vi "Set Start Command Val.vi"(8 "error in (no error)":errorcluster, 11 "Value":bool) -> (0 "error out":errorcluster)   [LabVIEW 2018, in "Outputs.lvlib"]
uses:
  Outputs.lvlib
  Public Controls/Specific Boolean Channel Write Data.ctl
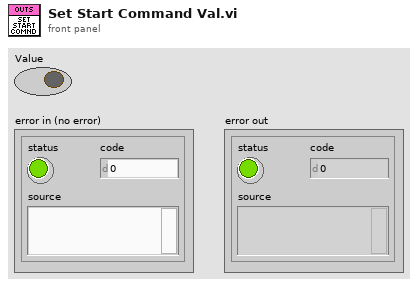
[diagram p1: front panel]
types:
  T1 = typedef "Outputs.lvlib/Specific Boolean Channel Write Data.ctl" = cluster{"Channel Index":i32, "Value":bool}
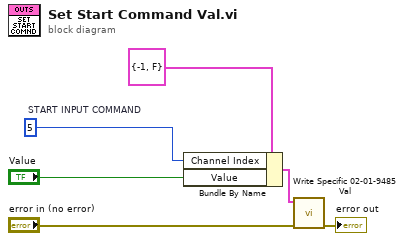
[diagram p0: block diagram]
diagram:
  w2 = 5  # START INPUT COMMAND
  n1 = Bundle By Name(cluster=T1 {"Channel Index"=-1, "Value"=FALSE} ("Chann and Val"), "Channel Index"=w2, "Value"="Value") -> (w1:T1)
  n2 = call "Write Specific 02-01-9485 Val.vi"("error in (no error)"="error in (no error)", "Chann and Val"=w1) -> ("error out"=→"error out":errorcluster)  [unwired: 9 in]
